vi "Countdown Timer FGV.vi"(8 "error in":errorcluster, 10 "Goal time":dbl, 11 "Action":T1=enum."Reset") -> (0 "error out":errorcluster, 1 "Time has elapsed?":bool, 2 "Time remaining (s)":dbl)   [LabVIEW 2018, in "Controller.lvlib"]
uses:
  Controller.lvlib
  ctl/Countdown Timer Action.ctl
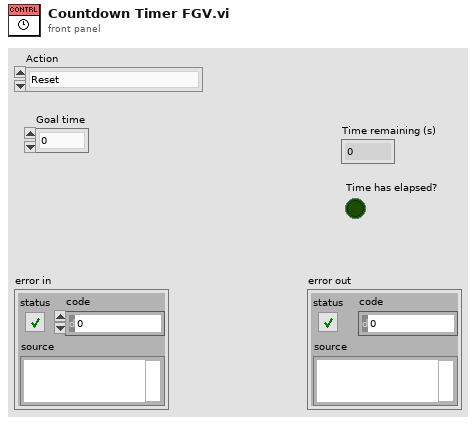
[diagram p1: front panel]
types:
  T1 = typedef "Controller.lvlib/Countdown Timer Action.ctl" = enum16{"Create (set goal time and start)", "Get (read)", "Reset"}
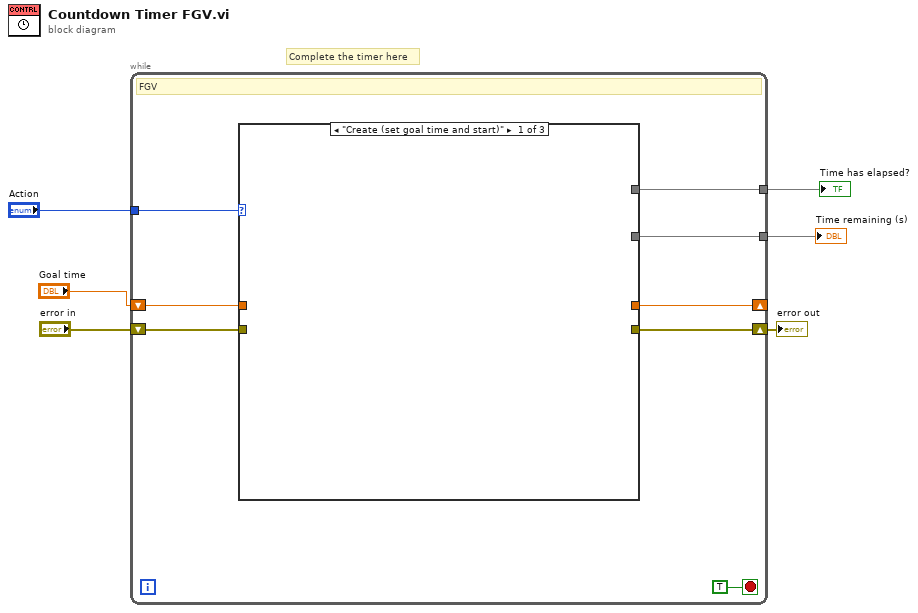
[diagram p0: block diagram]
diagram:
  # "Complete the timer here"
  n1 = while {
    tunnel: "Action" -> [w14]
    shift-right: [w11] -> w6
    shift-left: "error in" -> [w10]
    shift-right: [w12] -> _
    shift-left: "Goal time" -> [w9]
    tunnel: [w8] -> w2
    tunnel: [w7] -> w1
    stop <- TRUE stop-if-true
    # "FGV"
    n2 = case shown="\"Create (set goal time and start)\"" w14 {
      tunnel: [_ w16 _] -> w12
      tunnel: [_ w15 _] -> w11
      tunnel: w10 -> [_ w15 _]
      tunnel: w9 -> [_ w16 _]
      tunnel: [_ _ _] -> w8
      tunnel: [_ _ _] -> w7
      frame "Create (set goal time and start)" {
      }
      frame "Get (read)", Default {
      }
      frame "Reset" {
      }
    }
  }
  "error out" <- w6
  "Time has elapsed?" <- w1
  "Time remaining (s)" <- w2
